vi "setMainProperties.vi"(8 "error in (no error)":errorcluster, 10 "mainTextProperties":T1, 11 "TextDecoration in":refnum<class "TextDecoration.lvclass">) -> (0 "error out":errorcluster, 3 "TextDecoration out":refnum<class "TextDecoration.lvclass">)   [LabVIEW 2023, in "TLC_Scripto.lvlib" / "TextDecoration.lvclass"]
uses:
  TextDecoration.lvclass
  TextDecoration.lvclass/TextDecoration.ctl
  Ctrls/mainTextProperties.ctl
  TLC_Scripto.lvlib
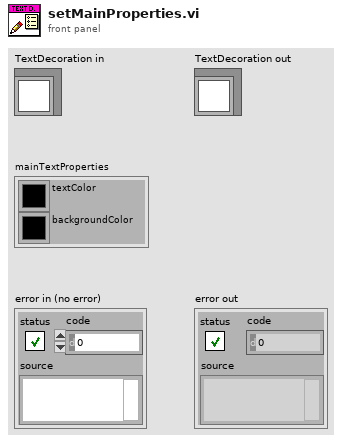
[diagram p1: front panel]
types:
  T1 = typedef "TLC_Scripto.lvlib/mainTextProperties.ctl" = cluster{"textColor":u32, "backgroundColor":u32}
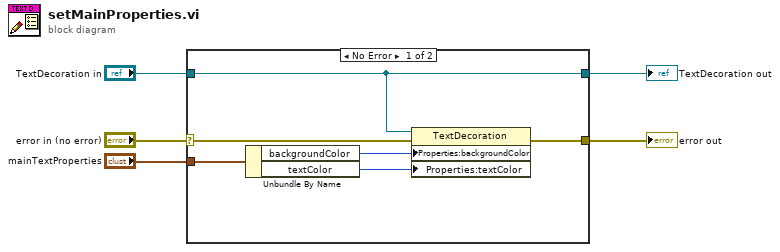
[diagram p0: block diagram]
diagram:
  n1 = case shown="No Error" "error in (no error)" {
    selector: "error in (no error)" -> [w7 w13]
    tunnel: [w6 w13] -> w4
    tunnel: [w11 w12] -> w2
    tunnel: "TextDecoration in" -> [w11 w12]
    tunnel: "mainTextProperties" -> [w10 _]
    frame No Error {
      n2 = Unbundle By Name(w10) -> ("backgroundColor"=w9:u32, "textColor"=w8:u32)
      n3 = property class="TextDecoration"(reference=w11, error in=w7, "Properties:backgroundColor"=w9, "Properties:textColor"=w8) -> (error out=w6:errorcluster)  [unwired: 1 out]
    }
    frame Error {
    }
  }
  "error out" <- w4
  "TextDecoration out" <- w2
